vi "SSL_set_mode.vi"(8 "error in (no error)":errorcluster, 10 "Mode":T1 items=["None"=0, "SSL_MODE_ENABLE_PARTIAL_WRITE"=1, "SSL_MODE_ACCEPT_MOVING_WRITE_BUFFER"=2, "SSL_MODE_AUTO_RETRY"=4, "SSL_MODE_RELEASE_BUFFERS"=16, "SSL_MODE_SEND_FALLBACK_SCSV"=128], 11 "SSL in":refnum<class "SSL.lvclass">) -> (0 "error out":errorcluster, 3 "SSL out":refnum<class "SSL.lvclass">)   [LabVIEW 2013, in "OpenSSL Socket.lvlib" / "SSL.lvclass"]
uses:
  SSL.lvclass
  SSL_Mode.ctl
  SSL-Lib/SSL-Lib.lvclass/SSL-Lib.ctl
  SSL.lvclass/SSL.ctl
  SSL-Lib/Read SSL Library Path.vi
  Read Handle.vi
  SSL-Lib/SSL-Lib.lvclass
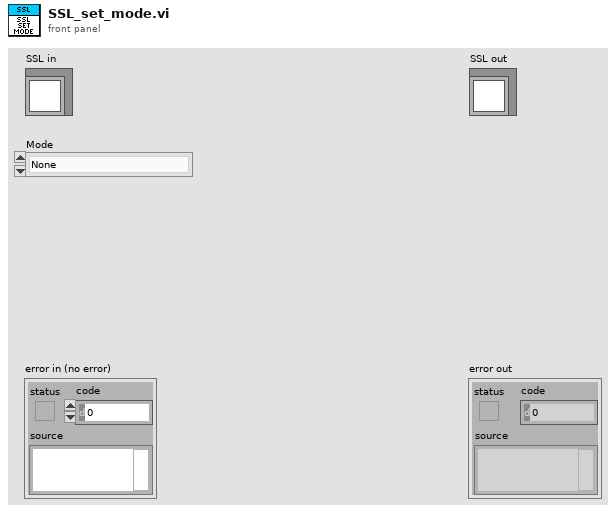
[diagram p1: front panel]
types:
  T1 = typedef "OpenSSL Socket.lvlib/SSL.lvclass/SSL_Mode.ctl" = i32
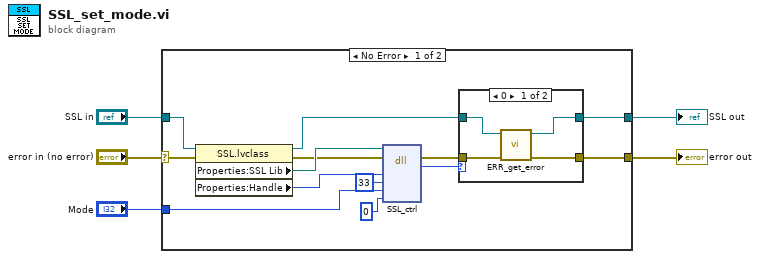
[diagram p0: block diagram]
diagram:
  n1 = case shown="No Error" "error in (no error)" {
    selector: "error in (no error)" -> [w14 w26]
    tunnel: [w10 w26] -> w4
    tunnel: [w8 w25] -> w2
    tunnel: "SSL in" -> [w15 w25]
    tunnel: "Mode" -> [w17 _]
    frame No Error {
      n2 = property class="SSL.lvclass"(reference=w15, error in=w14) -> (reference out=w9:refnum<class "SSL.lvclass">, error out=w6:errorcluster, "Properties:SSL Lib"=w12:path, "Properties:Handle"=w13:u64)
      n3 = dll-call lib="C:/Program Files (x86)/National Instruments/Shared/nissl/NIssleay32.dll" fn="SSL_ctrl"(path in=w12, error in=w6, "BIO"=w13, "cmd"=33, "larg"=w17, "parg"=u64 0 ("mode")) -> (error out=w11:errorcluster, "return type"=w7:i32)  [unwired: 5 in, 1 out]
      n4 = case shown="0" w7 {
        tunnel: w11 -> [w22 w24]
        tunnel: [w19 w24] -> w10
        tunnel: w9 -> [w21 w23]
        tunnel: [w20 w23] -> w8
        frame 0 {
          n5 = call "ERR_get_error.vi"("error in (no error)"=w22, "SSL-Lib in"=w21) -> ("error out"=w19:errorcluster, "SSL-Lib out"=w20:refnum<class "SSL.lvclass">)  [unwired: 8 in]
        }
        frame Default {
        }
      }
    }
    frame Error {
    }
  }
  "error out" <- w4
  "SSL out" <- w2
